vi "Convert MemberTable To Class.vi"(8 "error in (no error)":errorcluster, 10 "课程表":T1[][](array[typedef]), 11 "MemberTable in":refnum<class "TimeTable.lvclass">) -> (0 "error out":errorcluster, 3 "MemberTable out":refnum<class "TimeTable.lvclass">)   [LabVIEW 2015, in "TimeTable.lvclass"]
uses:
  TimeTable.lvclass
  Type Definitions/Table_Cell.ctl
  TimeTable.lvclass/TimeTable.ctl
panel:
  # "—"
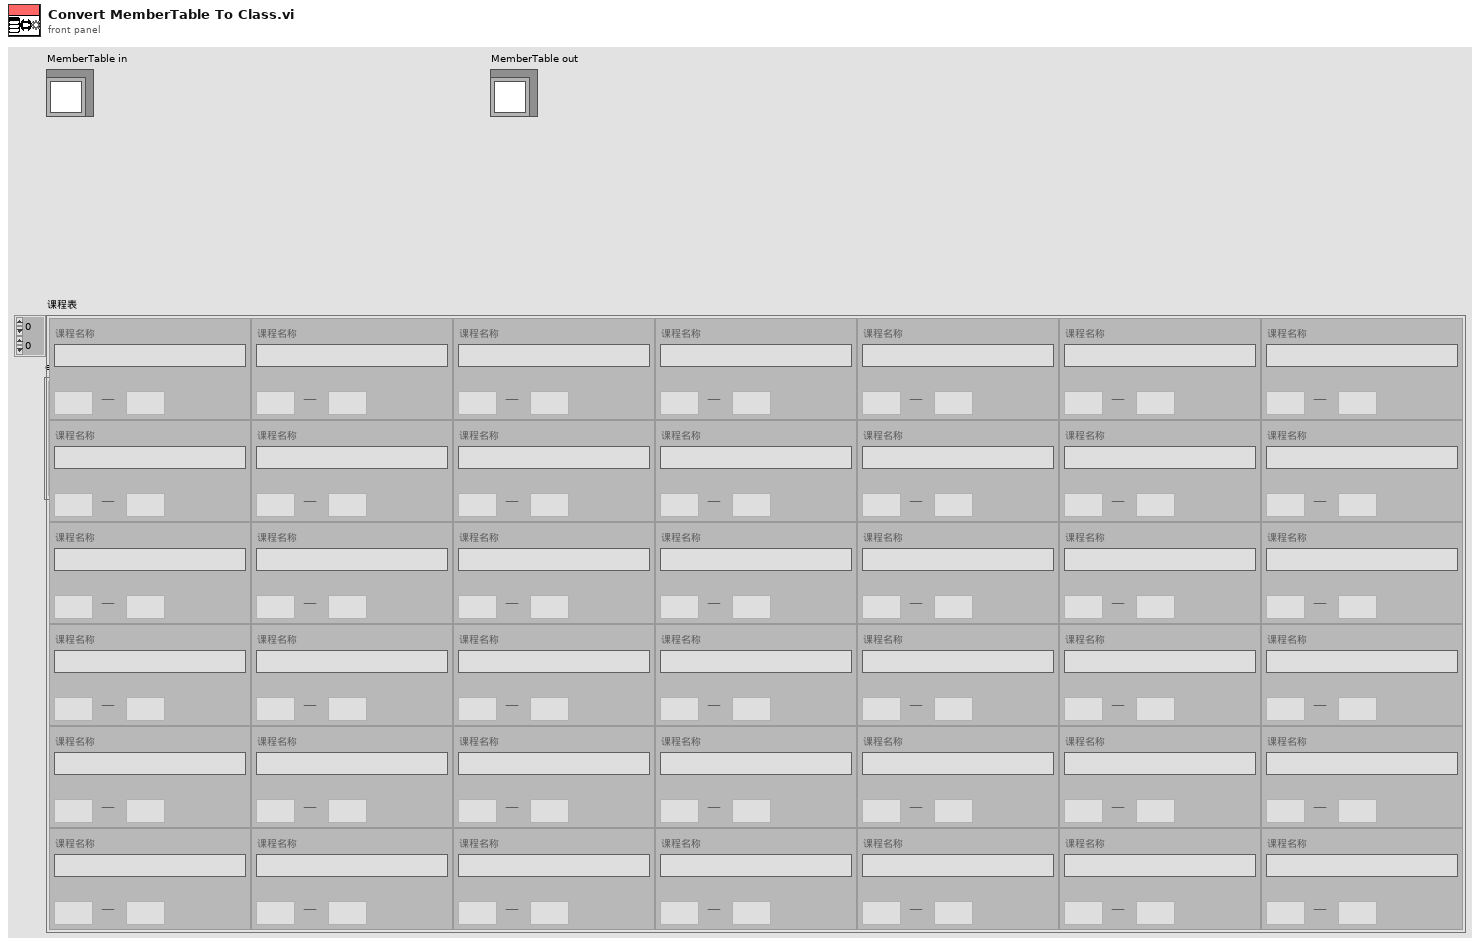
[diagram p1: front panel]
types:
  T1 = typedef "TimeTable.lvclass/Table_Cell.ctl" = cluster{"结束周":i32, "起始周":i32, "课程名称":string}
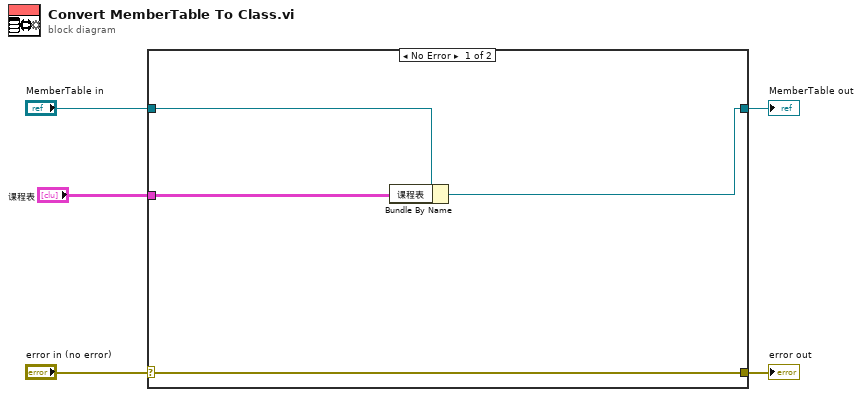
[diagram p0: block diagram]
diagram:
  n1 = case shown="No Error" "error in (no error)" {
    selector: "error in (no error)" -> [w9 w11]
    tunnel: [w9 w11] -> w4
    tunnel: [w6 w10] -> w2
    tunnel: "MemberTable in" -> [w8 w10]
    tunnel: "课程表" -> [w7 _]
    frame No Error {
      n2 = Bundle By Name(cluster=w8, "课程表"=w7) -> (w6:refnum<class "TimeTable.lvclass">)
    }
    frame Error {
    }
  }
  "error out" <- w4
  "MemberTable out" <- w2
